vi "HAPS_MCU_CMD_backup01.vi"(5 "HAPS_MCU_CMD":T3(ring), 7 "Tx/Rx":enum16{"Tx", "Rx"}(ring), 8 "error in":errorcluster, 10 "set_preamp":T1, 11 "set_ele":T2) -> (0 "error out":errorcluster)   [LabVIEW 2023, in "HAPS.lvlib"]
uses:
  HAPS.lvlib
panel:
  in  "Source":enum16{"MCU", "ACU"}(ring)
  in  "Enable?":enum16{"On", "OFF"}(ring)
  out "Time(ms)":dbl
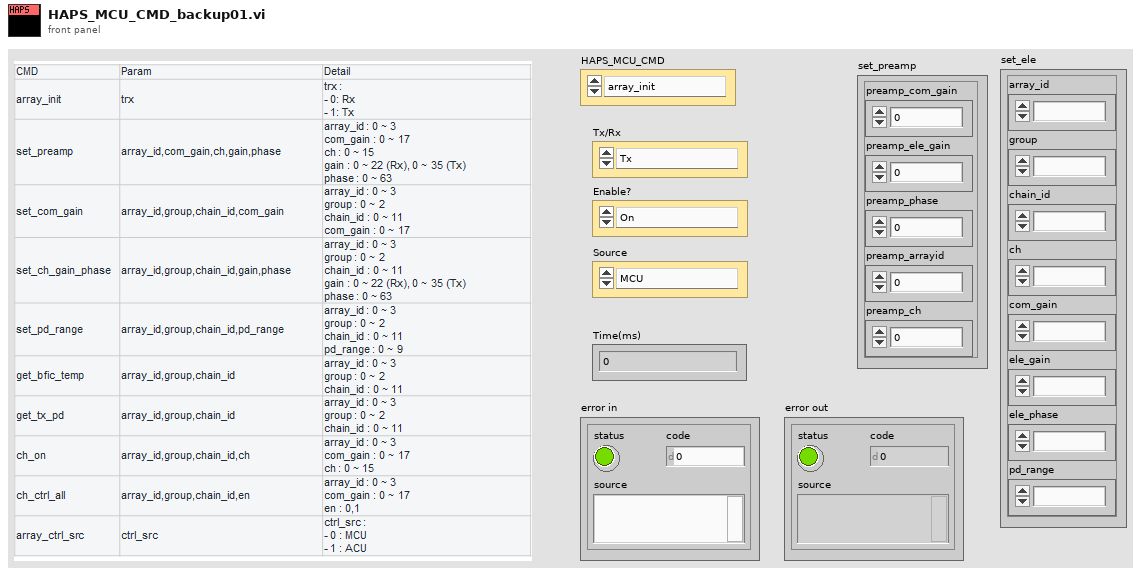
[diagram p1: front panel]
types:
  T1 = cluster{"preamp_arrayid":i32, "preamp_ch":i32, "preamp_com_gain":i32, "preamp_ele_gain":i32, "preamp_phase":i32}
  T2 = cluster{"ch":i32, "chain_id":i32, "group":i32, "array_id":i32, "ele_phase":i32, "ele_gain":i32, "com_gain":i32, "pd_range":i32}
  T3 = enum16{"array_init", "set_preamp", "set_com_gain", "set_ch_gain_phase", "set_pd_range", "get_preamp_temp", "get_bfic_temp", "get_tx_pd", "ch_on", "ch_ctrl_all", "array_ctrl_src"}
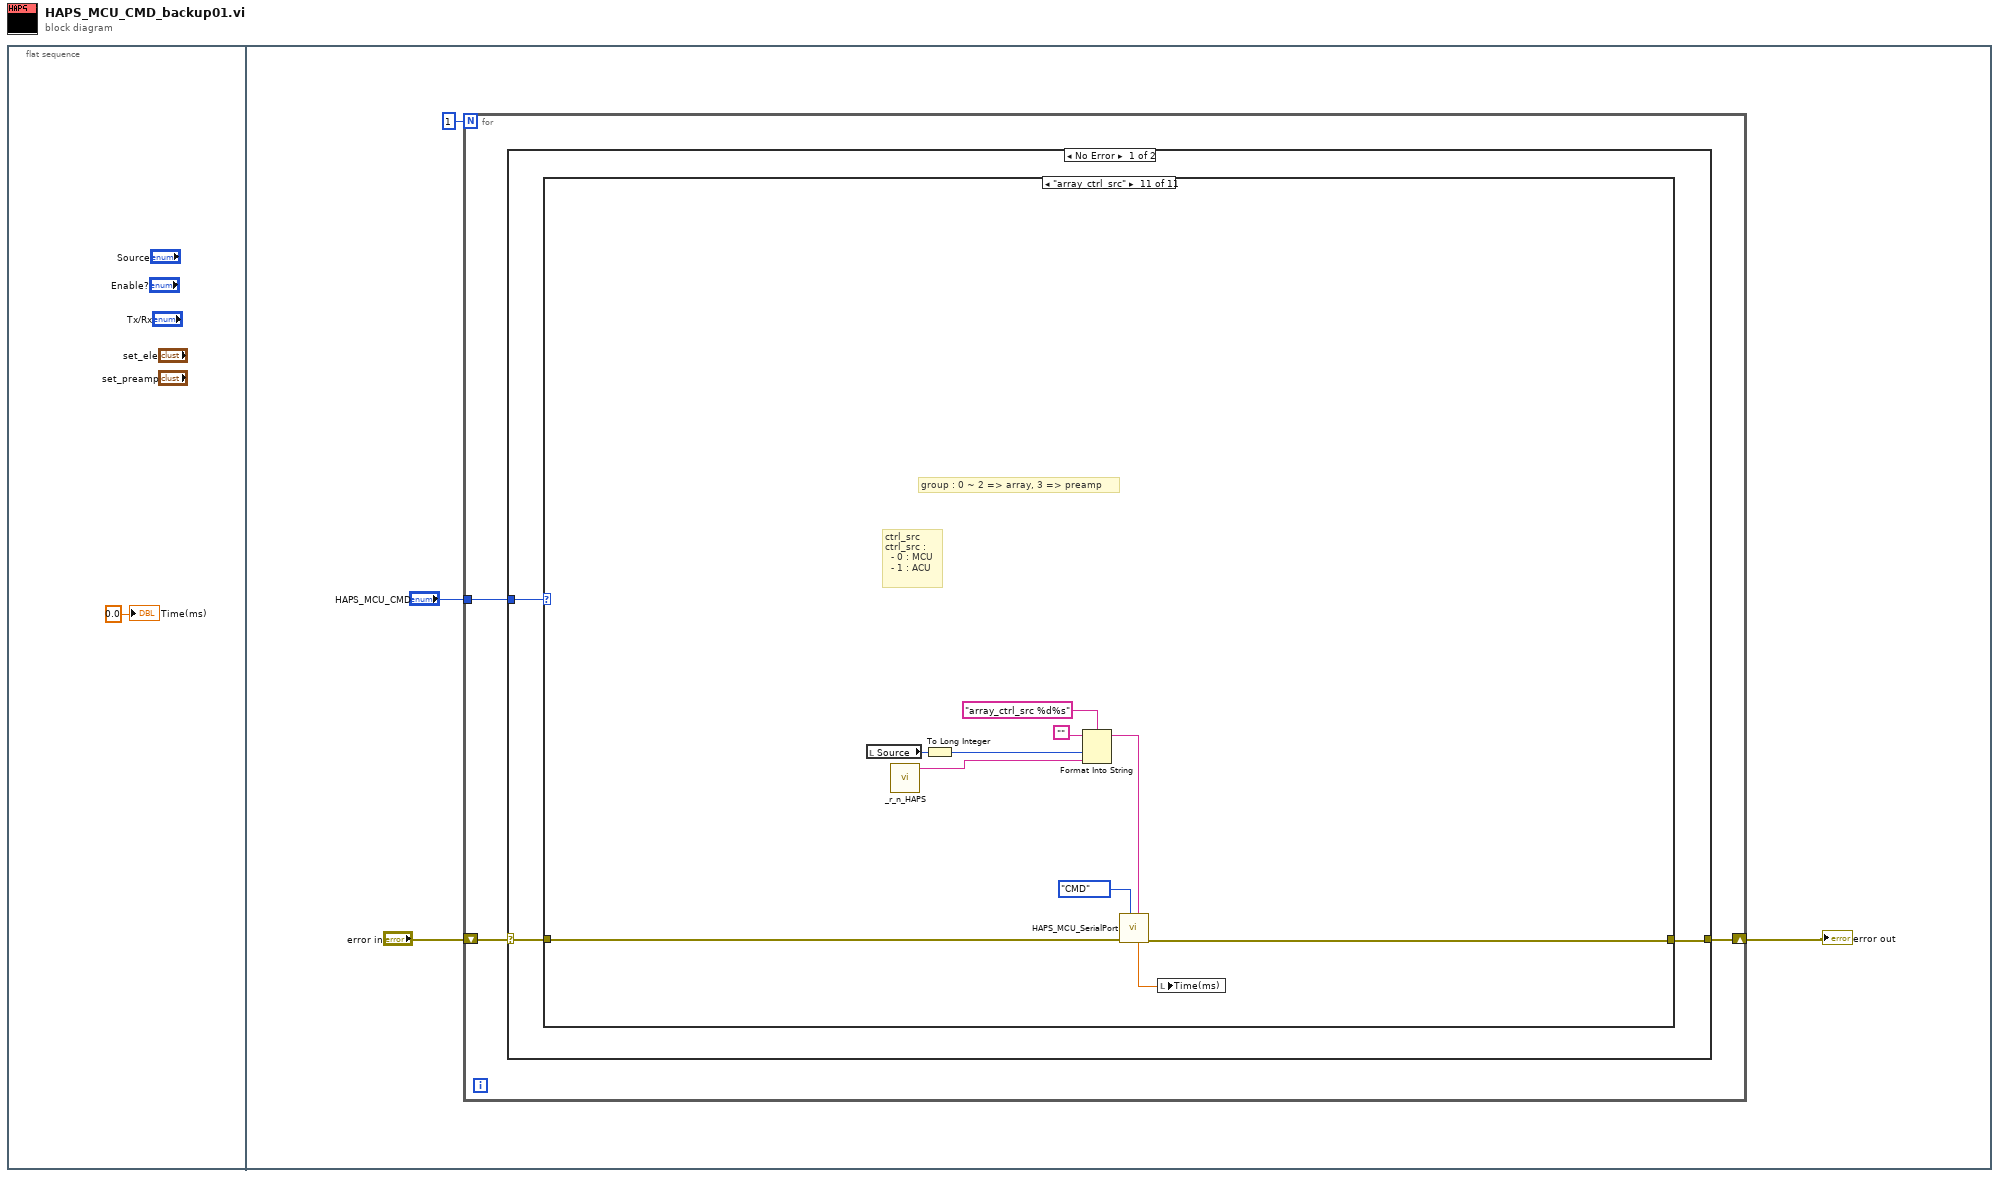
[diagram p0: block diagram]
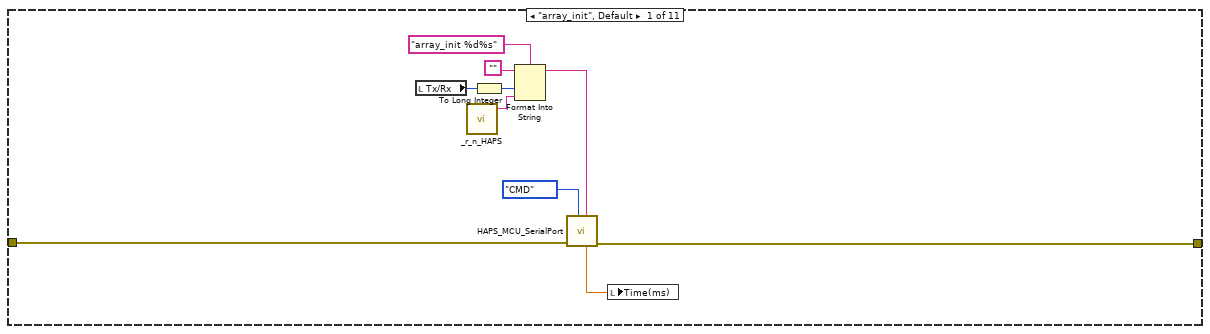
[diagram p2: hidden frame]
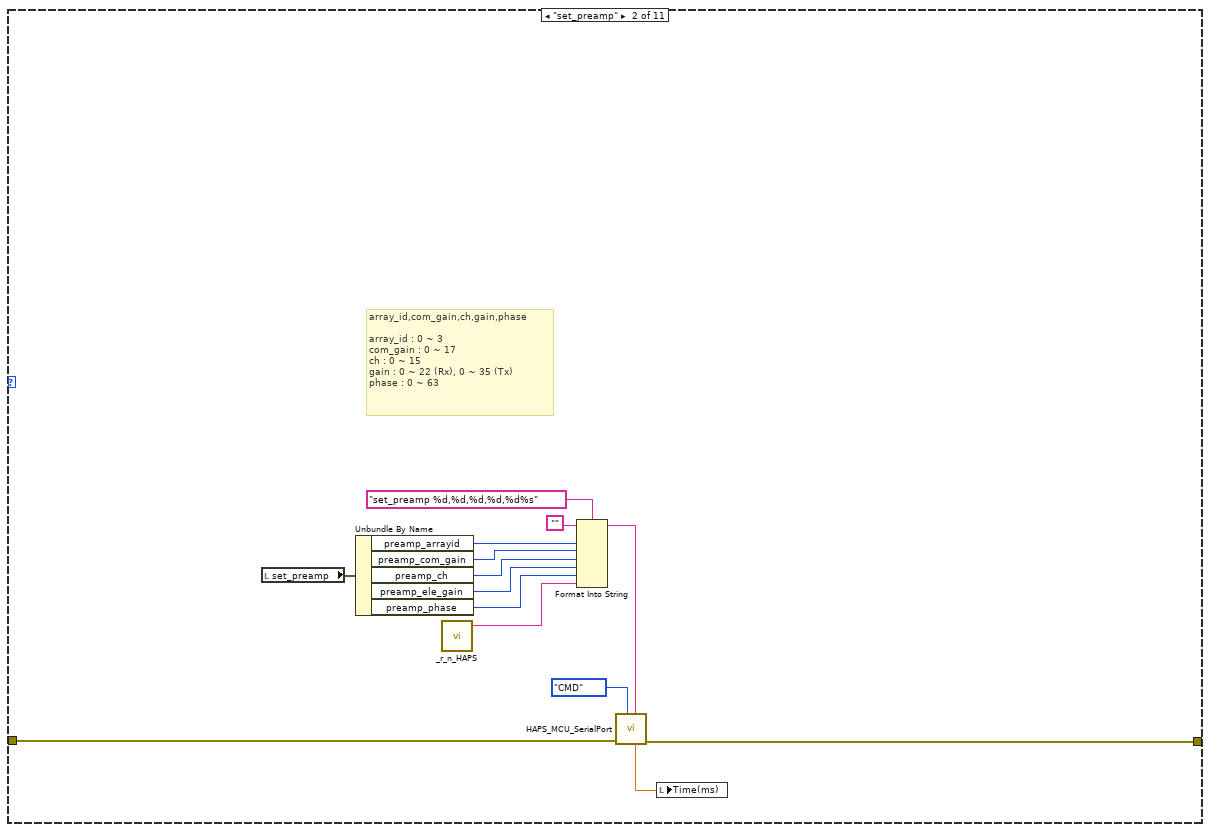
[diagram p3: hidden frame]
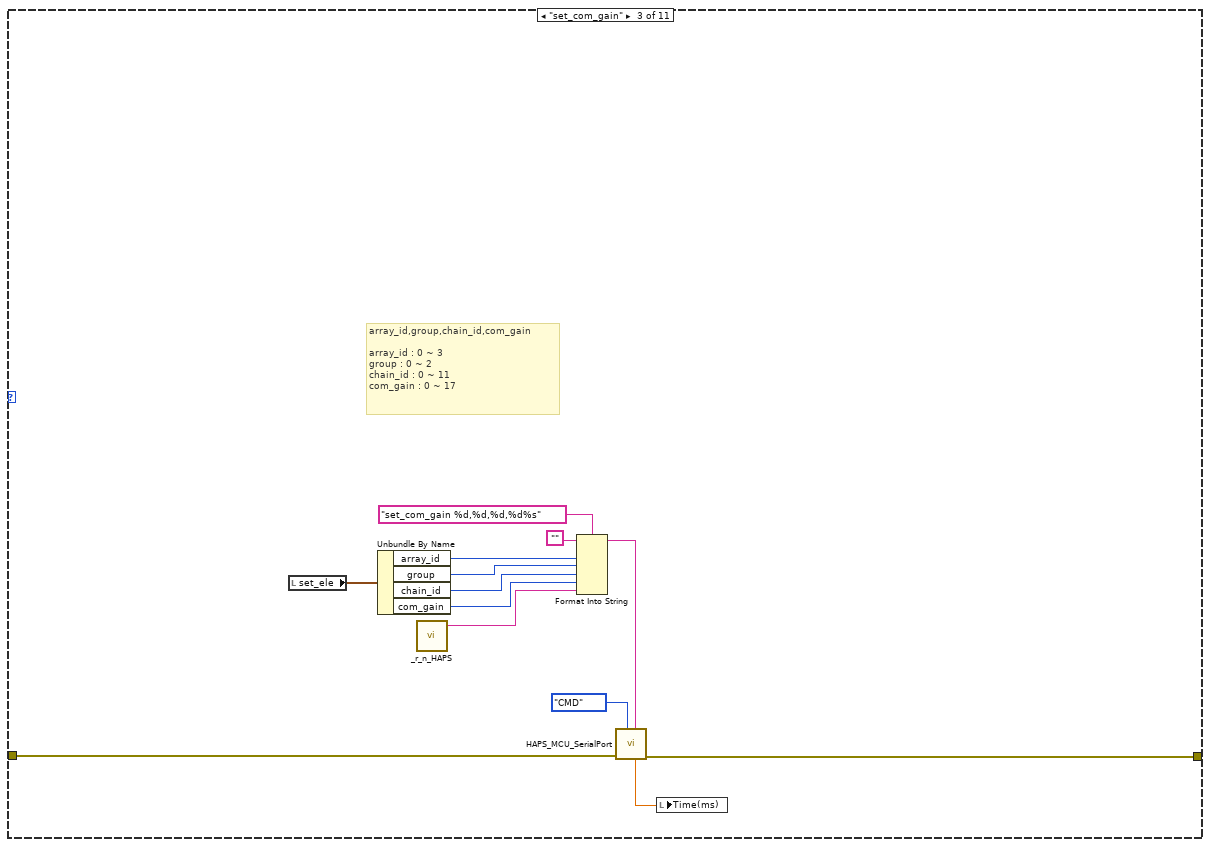
[diagram p4: hidden frame]
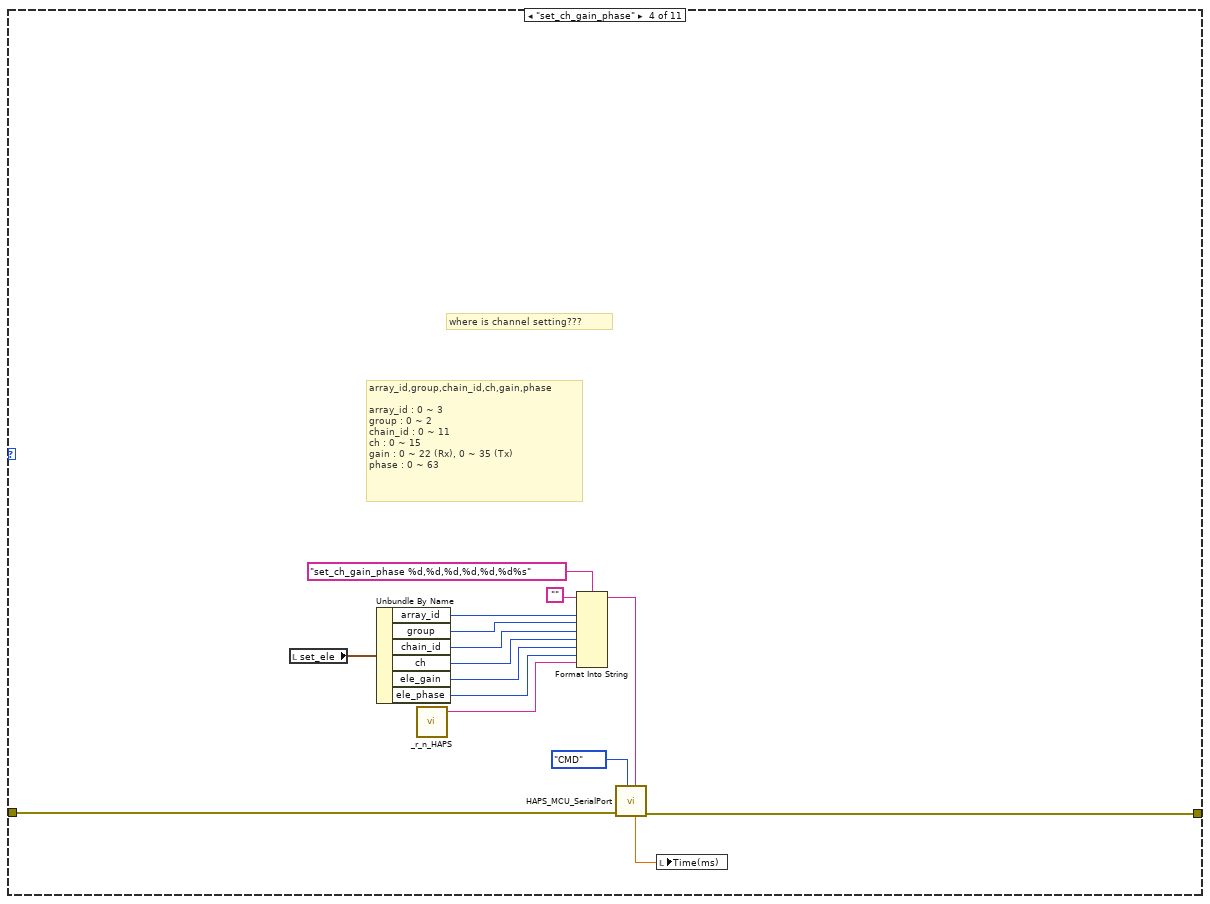
[diagram p5: hidden frame]
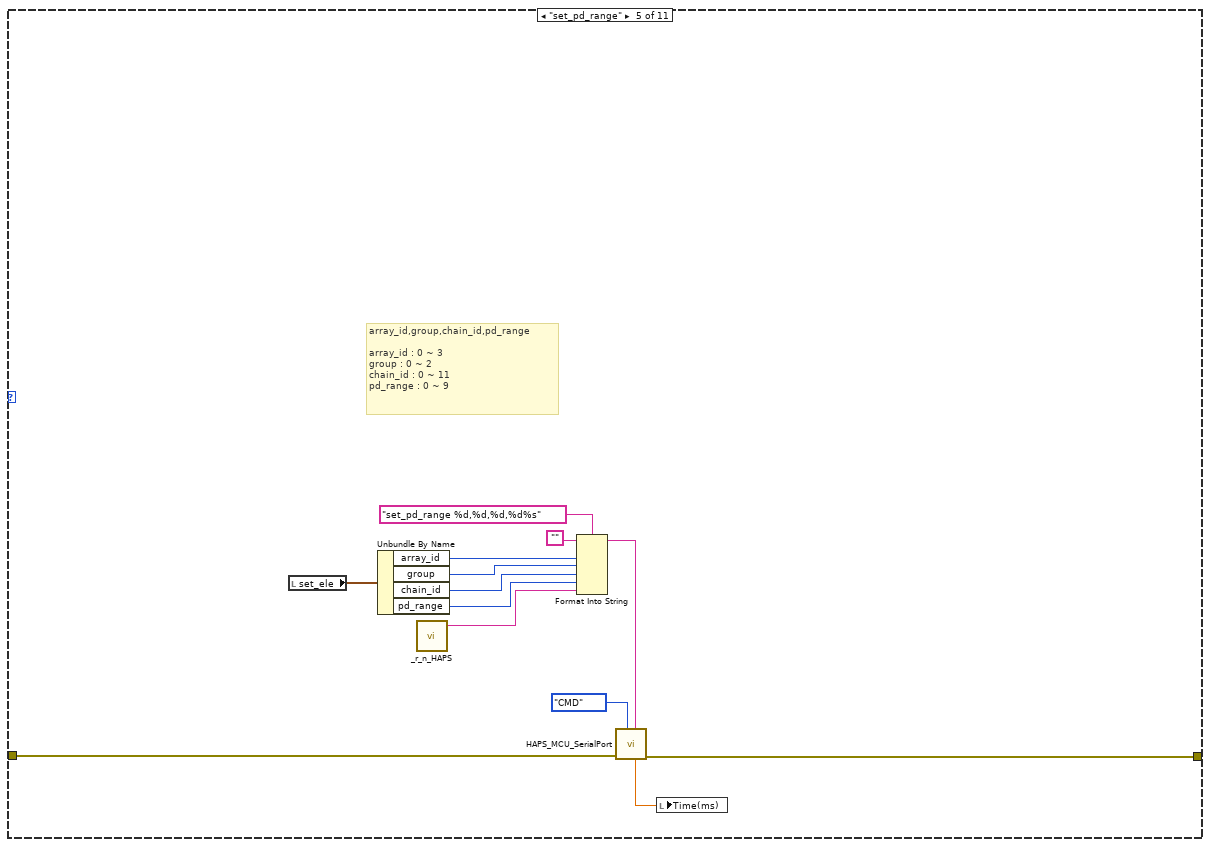
[diagram p6: hidden frame]
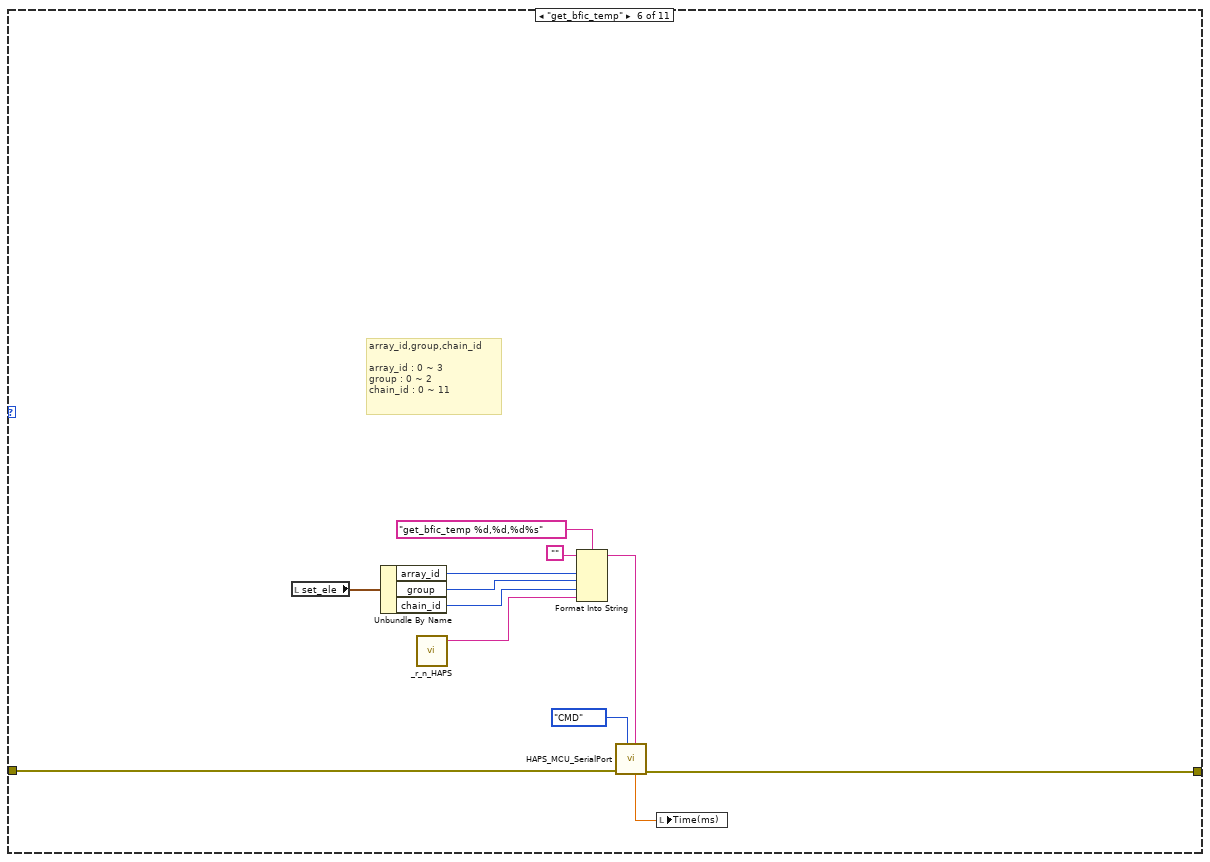
[diagram p7: hidden frame]
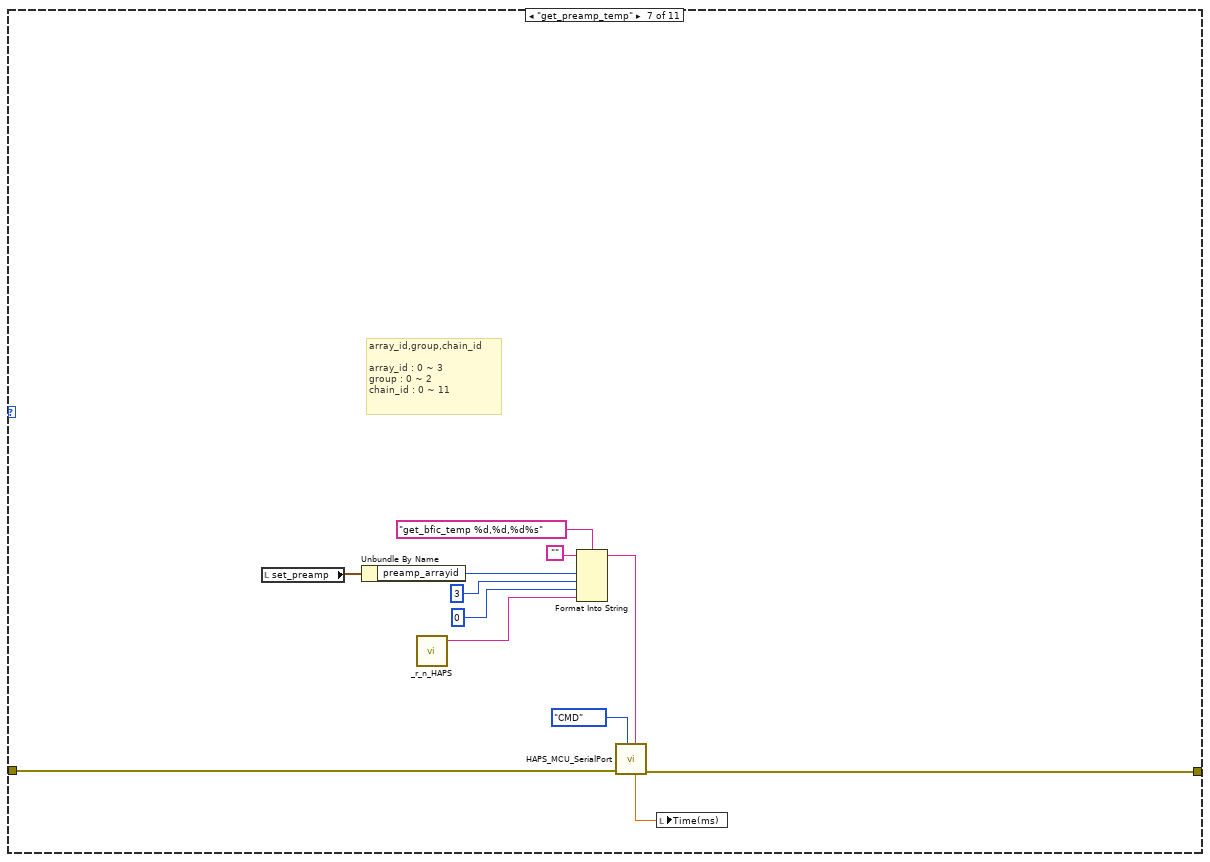
[diagram p8: hidden frame]
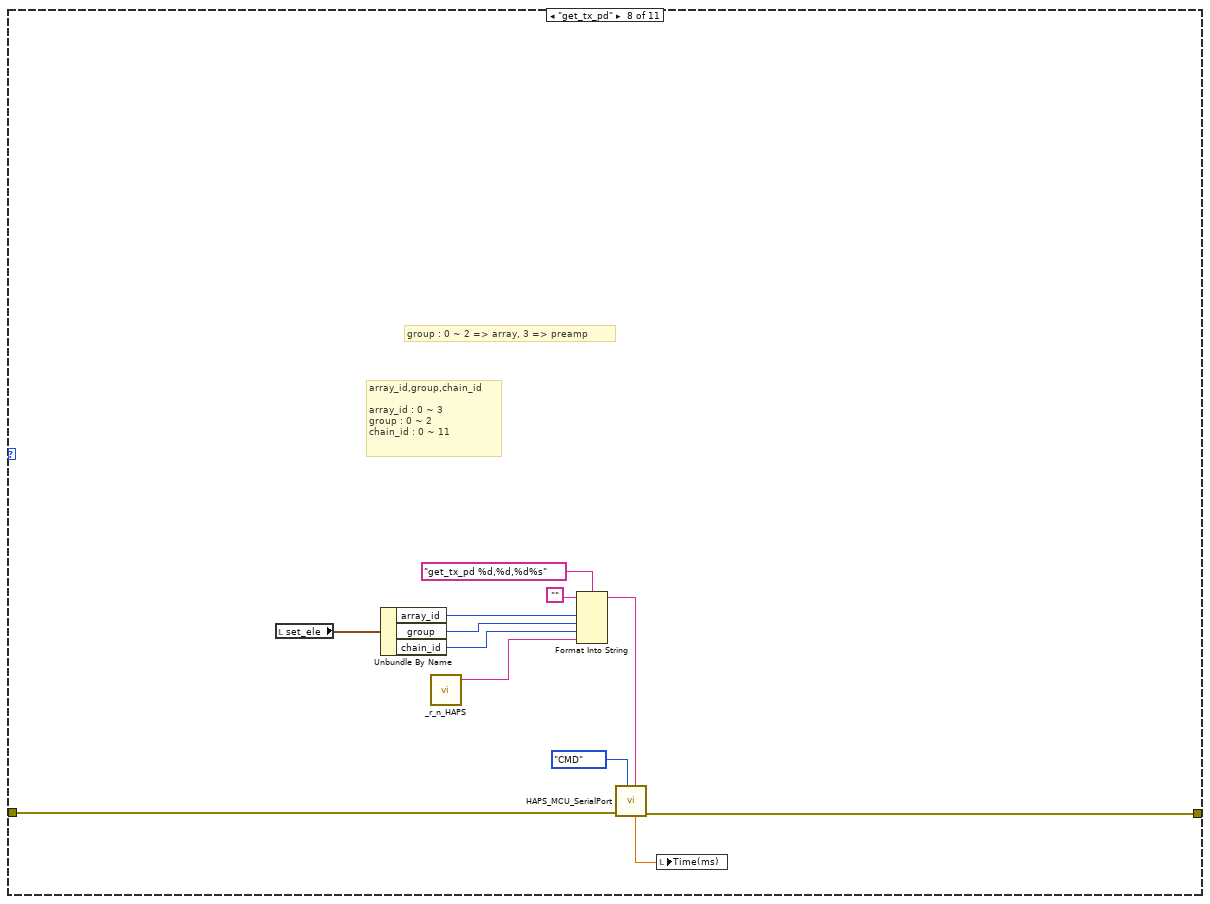
[diagram p9: hidden frame]
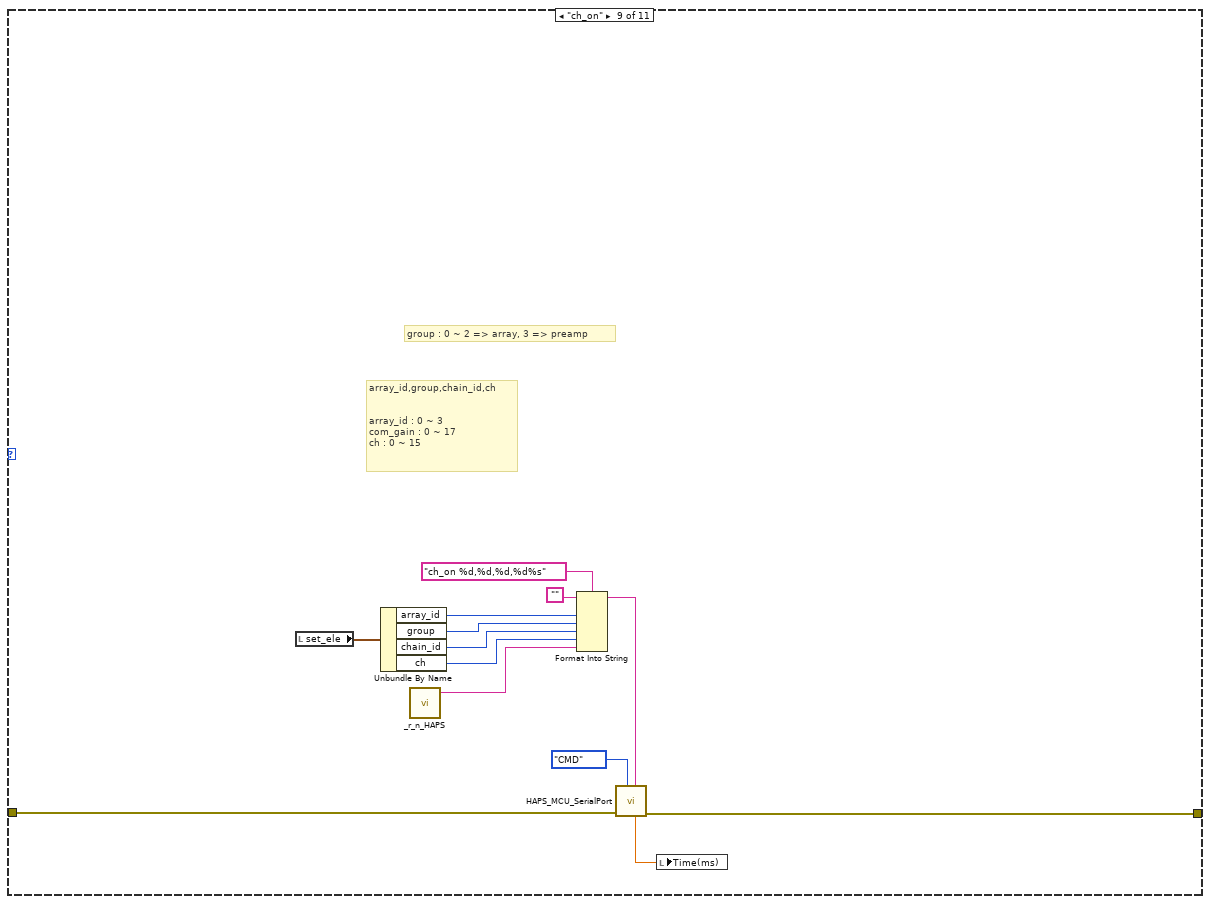
[diagram p10: hidden frame]
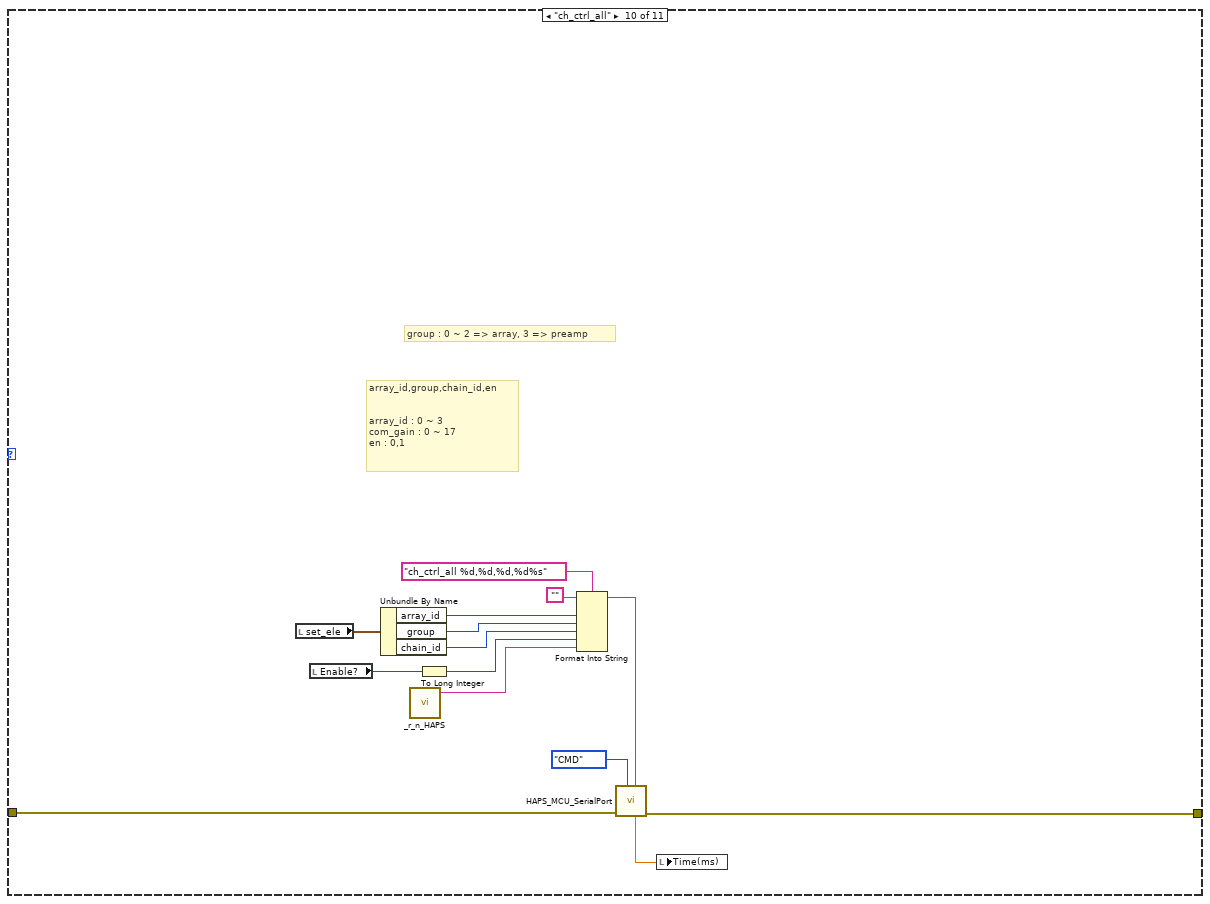
[diagram p11: hidden frame]
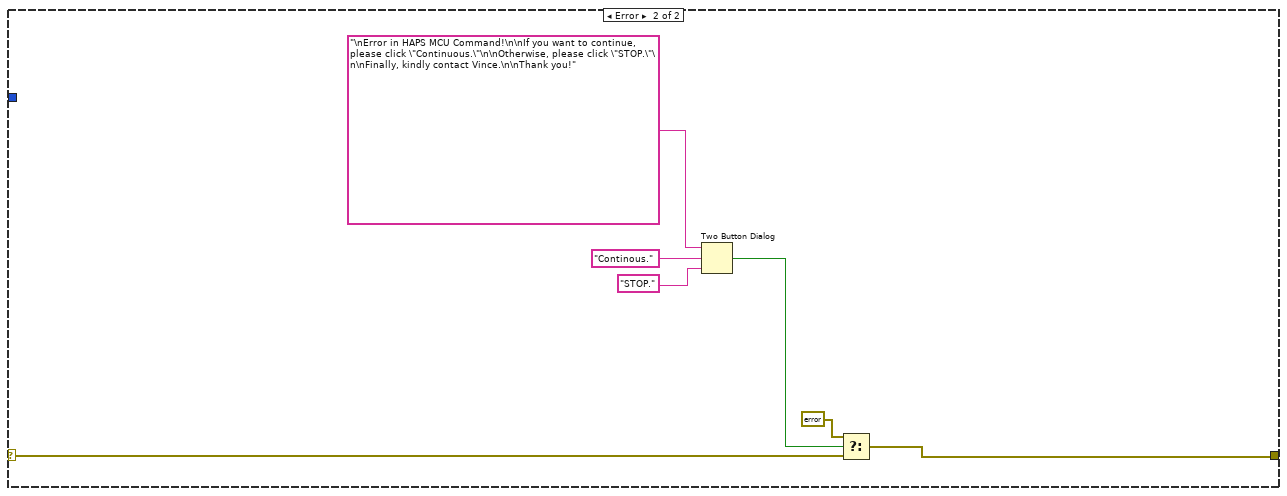
[diagram p12: hidden frame]
diagram:
  n1 = flat-sequence {
    frame #0 {
      "Time(ms)" <- 0.0 ("Time(ms)")
    }
    frame #1 {
      n2 = for {
        N: 1 -> [_]
        tunnel: "HAPS_MCU_CMD" -> [w6]
        shift-right: [w8] -> w2
        shift-left: "error in" -> [w7]
        n3 = case shown="No Error" w7 {
          selector: w7 -> [w11 w152]
          tunnel: [w9 w150] -> w8
          tunnel: w6 -> [w10 _]
          frame No Error {
            n4 = case shown="\"array_ctrl_src\"" w10 {
              tunnel: w11 -> [w21 w35 w48 w63 w76 w88 w100 w112 w125 w139 w149]
              tunnel: [w20 w34 w47 w62 w75 w87 w99 w111 w124 w138 w148] -> w9
              frame "array_init", Default {
                n5 = local read "Tx/Rx"() -> (w15:enum16{"Tx", "Rx"})
                n6 = call "_r_n_HAPS.vi"() -> ("command"=w13:string)  [unwired: 5 in]
                n7 = To Long Integer(number=w15) -> (32bit integer=w14:i32)
                n8 = Format Into String(format string="array_init %d%s" ("Command"), initial string="", w14, w13) -> (resulting string=w12:string)  [unwired: 1 in, 1 out]
                n9 = call "HAPS_MCU_SerialPort.vi"("Command"=w12, "HAPS_SerialPort_Func"=enum16{"Init", "Close", "CMD"}."CMD" ("HAPS_SerialPort"), "error in"=w21) -> ("error out"=w20:errorcluster, "Time(ms)"=w19:dbl)  [unwired: 6 in, 1 out]
                n10 = local write "Time(ms)"(w19) -> ()
              }
              frame "set_preamp" {
                # "array_id,com_gain,ch,gain,phase\n\narray_id : 0 ~ 3\ncom_gain : 0 ~ 17\nch : 0 ~ 15\ngain : 0 ~ 22 (Rx), 0 ~ 35 (Tx)\nphase : 0 ~ 63"
                n11 = local read "set_preamp"() -> (w27:T1)
                n12 = Unbundle By Name(w27) -> ("preamp_arrayid"=w28:i32, "preamp_com_gain"=w26:i32, "preamp_ch"=w25:i32, "preamp_ele_gain"=w24:i32, "preamp_phase"=w23:i32)
                n13 = call "_r_n_HAPS.vi"() -> ("command"=w22:string)  [unwired: 5 in]
                n14 = Format Into String(format string="set_preamp %d,%d,%d,%d,%d%s" ("Command"), initial string="", w28, w26, w25, w24, w23, w22) -> (resulting string=w29:string)  [unwired: 1 in, 1 out]
                n15 = call "HAPS_MCU_SerialPort.vi"("Command"=w29, "HAPS_SerialPort_Func"=enum16{"Init", "Close", "CMD"}."CMD" ("HAPS_SerialPort"), "error in"=w35) -> ("error out"=w34:errorcluster, "Time(ms)"=w33:dbl)  [unwired: 6 in, 1 out]
                n16 = local write "Time(ms)"(w33) -> ()
              }
              frame "set_com_gain" {
                # "array_id,group,chain_id,com_gain\n\narray_id : 0 ~ 3\ngroup : 0 ~ 2\nchain_id : 0 ~ 11\ncom_gain : 0 ~ 17"
                n17 = local read "set_ele"() -> (w37:T2)
                n18 = Unbundle By Name(w37) -> ("array_id"=w41:i32, "group"=w40:i32, "chain_id"=w39:i32, "com_gain"=w38:i32)
                n19 = call "_r_n_HAPS.vi"() -> ("command"=w36:string)  [unwired: 5 in]
                n20 = Format Into String(format string="set_com_gain %d,%d,%d,%d%s" ("Command"), initial string="", w41, w40, w39, w38, w36) -> (resulting string=w42:string)  [unwired: 1 in, 1 out]
                n21 = call "HAPS_MCU_SerialPort.vi"("Command"=w42, "HAPS_SerialPort_Func"=enum16{"Init", "Close", "CMD"}."CMD" ("HAPS_SerialPort"), "error in"=w48) -> ("error out"=w47:errorcluster, "Time(ms)"=w46:dbl)  [unwired: 6 in, 1 out]
                n22 = local write "Time(ms)"(w46) -> ()
              }
              frame "set_ch_gain_phase" {
                # "where is channel setting???"
                # "array_id,group,chain_id,ch,gain,phase\n\narray_id : 0 ~ 3\ngroup : 0 ~ 2\nchain_id : 0 ~ 11\nch : 0 ~ 15\ngain : 0 ~ 22 (Rx), 0 ~ 35 (Tx)\nphase : 0 ~ 63"
                n23 = local read "set_ele"() -> (w52:T2)
                n24 = Unbundle By Name(w52) -> ("array_id"=w56:i32, "group"=w55:i32, "chain_id"=w54:i32, "ch"=w53:i32, "ele_gain"=w51:i32, "ele_phase"=w50:i32)
                n25 = call "_r_n_HAPS.vi"() -> ("command"=w49:string)  [unwired: 5 in]
                n26 = Format Into String(format string="set_ch_gain_phase %d,%d,%d,%d,%d,%d%s" ("Command"), initial string="", w56, w55, w54, w53, w51, w50, w49) -> (resulting string=w57:string)  [unwired: 1 in, 1 out]
                n27 = call "HAPS_MCU_SerialPort.vi"("Command"=w57, "HAPS_SerialPort_Func"=enum16{"Init", "Close", "CMD"}."CMD" ("HAPS_SerialPort"), "error in"=w63) -> ("error out"=w62:errorcluster, "Time(ms)"=w61:dbl)  [unwired: 6 in, 1 out]
                n28 = local write "Time(ms)"(w61) -> ()
              }
              frame "set_pd_range" {
                # "array_id,group,chain_id,pd_range\n\narray_id : 0 ~ 3\ngroup : 0 ~ 2\nchain_id : 0 ~ 11\npd_range : 0 ~ 9"
                n29 = local read "set_ele"() -> (w65:T2)
                n30 = Unbundle By Name(w65) -> ("array_id"=w69:i32, "group"=w68:i32, "chain_id"=w67:i32, "pd_range"=w66:i32)
                n31 = call "_r_n_HAPS.vi"() -> ("command"=w64:string)  [unwired: 5 in]
                n32 = Format Into String(format string="set_pd_range %d,%d,%d,%d%s" ("Command"), initial string="", w69, w68, w67, w66, w64) -> (resulting string=w70:string)  [unwired: 1 in, 1 out]
                n33 = call "HAPS_MCU_SerialPort.vi"("Command"=w70, "HAPS_SerialPort_Func"=enum16{"Init", "Close", "CMD"}."CMD" ("HAPS_SerialPort"), "error in"=w76) -> ("error out"=w75:errorcluster, "Time(ms)"=w74:dbl)  [unwired: 6 in, 1 out]
                n34 = local write "Time(ms)"(w74) -> ()
              }
              frame "get_bfic_temp" {
                # "array_id,group,chain_id\n\narray_id : 0 ~ 3\ngroup : 0 ~ 2\nchain_id : 0 ~ 11"
                n35 = local read "set_ele"() -> (w78:T2)
                n36 = Unbundle By Name(w78) -> ("array_id"=w81:i32, "group"=w80:i32, "chain_id"=w79:i32)
                n37 = call "_r_n_HAPS.vi"() -> ("command"=w77:string)  [unwired: 5 in]
                n38 = Format Into String(format string="get_bfic_temp %d,%d,%d%s" ("Command"), initial string="", w81, w80, w79, w77) -> (resulting string=w82:string)  [unwired: 1 in, 1 out]
                n39 = call "HAPS_MCU_SerialPort.vi"("Command"=w82, "HAPS_SerialPort_Func"=enum16{"Init", "Close", "CMD"}."CMD" ("HAPS_SerialPort"), "error in"=w88) -> ("error out"=w87:errorcluster, "Time(ms)"=w86:dbl)  [unwired: 6 in, 1 out]
                n40 = local write "Time(ms)"(w86) -> ()
              }
              frame "get_preamp_temp" {
                # "array_id,group,chain_id\n\narray_id : 0 ~ 3\ngroup : 0 ~ 2\nchain_id : 0 ~ 11"
                n41 = local read "set_preamp"() -> (w91:T1)
                n42 = Unbundle By Name(w91) -> ("preamp_arrayid"=w93:i32)
                n43 = call "_r_n_HAPS.vi"() -> ("command"=w92:string)  [unwired: 5 in]
                n44 = Format Into String(format string="get_bfic_temp %d,%d,%d%s" ("Command"), initial string="", w93, 3 ("input 2"), 0 ("input 3"), w92) -> (resulting string=w94:string)  [unwired: 1 in, 1 out]
                n45 = call "HAPS_MCU_SerialPort.vi"("Command"=w94, "HAPS_SerialPort_Func"=enum16{"Init", "Close", "CMD"}."CMD" ("HAPS_SerialPort"), "error in"=w100) -> ("error out"=w99:errorcluster, "Time(ms)"=w98:dbl)  [unwired: 6 in, 1 out]
                n46 = local write "Time(ms)"(w98) -> ()
              }
              frame "get_tx_pd" {
                # "group : 0 ~ 2 => array, 3 => preamp"
                # "array_id,group,chain_id\n\narray_id : 0 ~ 3\ngroup : 0 ~ 2\nchain_id : 0 ~ 11"
                n47 = local read "set_ele"() -> (w103:T2)
                n48 = Unbundle By Name(w103) -> ("array_id"=w105:i32, "group"=w102:i32, "chain_id"=w101:i32)
                n49 = call "_r_n_HAPS.vi"() -> ("command"=w104:string)  [unwired: 5 in]
                n50 = Format Into String(format string="get_tx_pd %d,%d,%d%s" ("Command"), initial string="", w105, w102, w101, w104) -> (resulting string=w106:string)  [unwired: 1 in, 1 out]
                n51 = call "HAPS_MCU_SerialPort.vi"("Command"=w106, "HAPS_SerialPort_Func"=enum16{"Init", "Close", "CMD"}."CMD" ("HAPS_SerialPort"), "error in"=w112) -> ("error out"=w111:errorcluster, "Time(ms)"=w110:dbl)  [unwired: 6 in, 1 out]
                n52 = local write "Time(ms)"(w110) -> ()
              }
              frame "ch_on" {
                # "group : 0 ~ 2 => array, 3 => preamp"
                # "array_id,group,chain_id,ch\n\n\narray_id : 0 ~ 3\ncom_gain : 0 ~ 17\nch : 0 ~ 15"
                n53 = local read "set_ele"() -> (w117:T2)
                n54 = Unbundle By Name(w117) -> ("array_id"=w118:i32, "group"=w116:i32, "chain_id"=w115:i32, "ch"=w114:i32)
                n55 = call "_r_n_HAPS.vi"() -> ("command"=w113:string)  [unwired: 5 in]
                n56 = Format Into String(format string="ch_on %d,%d,%d,%d%s" ("Command"), initial string="", w118, w116, w115, w114, w113) -> (resulting string=w119:string)  [unwired: 1 in, 1 out]
                n57 = call "HAPS_MCU_SerialPort.vi"("Command"=w119, "HAPS_SerialPort_Func"=enum16{"Init", "Close", "CMD"}."CMD" ("HAPS_SerialPort"), "error in"=w125) -> ("error out"=w124:errorcluster, "Time(ms)"=w123:dbl)  [unwired: 6 in, 1 out]
                n58 = local write "Time(ms)"(w123) -> ()
              }
              frame "ch_ctrl_all" {
                # "group : 0 ~ 2 => array, 3 => preamp"
                # "array_id,group,chain_id,en\n\n\narray_id : 0 ~ 3\ncom_gain : 0 ~ 17\nen : 0,1"
                n59 = local read "set_ele"() -> (w131:T2)
                n60 = local read "Enable?"() -> (w127:enum16{"On", "OFF"})
                n61 = Unbundle By Name(w131) -> ("array_id"=w132:i32, "group"=w130:i32, "chain_id"=w129:i32)
                n62 = call "_r_n_HAPS.vi"() -> ("command"=w128:string)  [unwired: 5 in]
                n63 = To Long Integer(number=w127) -> (32bit integer=w126:i32)
                n64 = Format Into String(format string="ch_ctrl_all %d,%d,%d,%d%s" ("Command"), initial string="", w132, w130, w129, w126, w128) -> (resulting string=w133:string)  [unwired: 1 in, 1 out]
                n65 = call "HAPS_MCU_SerialPort.vi"("Command"=w133, "HAPS_SerialPort_Func"=enum16{"Init", "Close", "CMD"}."CMD" ("HAPS_SerialPort"), "error in"=w139) -> ("error out"=w138:errorcluster, "Time(ms)"=w137:dbl)  [unwired: 6 in, 1 out]
                n66 = local write "Time(ms)"(w137) -> ()
              }
              frame "array_ctrl_src" {
                # "group : 0 ~ 2 => array, 3 => preamp"
                # "ctrl_src\nctrl_src : \n  - 0 : MCU\n  - 1 : ACU"
                n67 = local read "Source"() -> (w142:enum16{"MCU", "ACU"})
                n68 = call "_r_n_HAPS.vi"() -> ("command"=w140:string)  [unwired: 5 in]
                n69 = To Long Integer(number=w142) -> (32bit integer=w141:i32)
                n70 = Format Into String(format string="array_ctrl_src %d%s" ("Command"), initial string="", w141, w140) -> (resulting string=w143:string)  [unwired: 1 in, 1 out]
                n71 = call "HAPS_MCU_SerialPort.vi"("Command"=w143, "HAPS_SerialPort_Func"=enum16{"Init", "Close", "CMD"}."CMD" ("HAPS_SerialPort"), "error in"=w149) -> ("error out"=w148:errorcluster, "Time(ms)"=w147:dbl)  [unwired: 6 in, 1 out]
                n72 = local write "Time(ms)"(w147) -> ()
              }
            }
          }
          frame Error {
            n73 = Two Button Dialog(message="\nError in HAPS MCU Command!\n\nIf you want to continue, please click \"Continuous.\"\n\nOtherwise, please click \"STOP.\"\n\nFinally, kindly contact Vince.\n\nThank you!", 1:"STOP." ("F button name (\"Cancel\")"), 2:"Continous." ("T button name (\"OK\")")) -> (T button?=w153:bool)
            n74 = Select(t=errorcluster {"status"=FALSE, "code"=0, "source"=""}, s=w153, f=w152) -> (s? t:f=w150:errorcluster)
          }
        }
      }
      "error out" <- w2
    }
  }
